vi "filename.vi"(8 "Filename":string="LabVIEW Data", 11 "Pasta Destino":path) -> (3 "filename output":path)   [LabVIEW 2018]
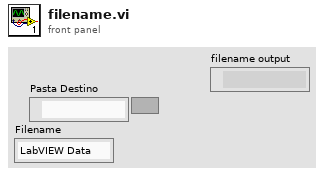
[diagram p1: front panel]
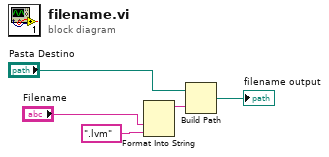
[diagram p0: block diagram]
diagram:
  n1 = Format Into String("Filename", ".lvm") -> (resulting string=w4:string)  [unwired: 3 in, 1 out]
  n2 = Build Path(base path="Pasta Destino", name or relative path=w4) -> (appended path=→"filename output":path)
